vi "UpdateActualDepsList.vi"(8 "error in (no error)":errorcluster, 10 "UpdateForChangedLibrariesOnly":bool=TRUE, 11 "Workspace Path":path=path "C:/sw-deps-monitor") -> (0 "error out":errorcluster)   [LabVIEW 2019, in "Hawkeye.lvlib"]
uses:
  Hawkeye.lvlib
  <vilib>/Wiresmith Technology/G CLI/CLI Class/CLI.lvclass
  <vilib>/SLL Toolkit/SLL String/SLL String.lvlib
panel:
  in  "GUI Mode? {F)":bool
  in  "Tab Control":enum32{"GUI Mode", "CLI Mode"}(tab)
  out "Args":string[](array[string])=["C:\\sw-deps-monitor", "True"]
  out "Status Indicator":string
  # "When in GUI Mode, the controls will be used, \nIn CLI Mode, the Args will be used"
  # "Workspace Path"
  # "UpdateChangedLibsOnly? True/False"
  # "Command to run the VI from terminal\ng-cli -v --lv-ver 2023 --arch 32 \"C:\\sw-deps-monitor\\CICD\\AutomatedChecks\\UpdateActualDepsList.vi\" -- \"C:\\sw-deps-monitor\" \"False\""
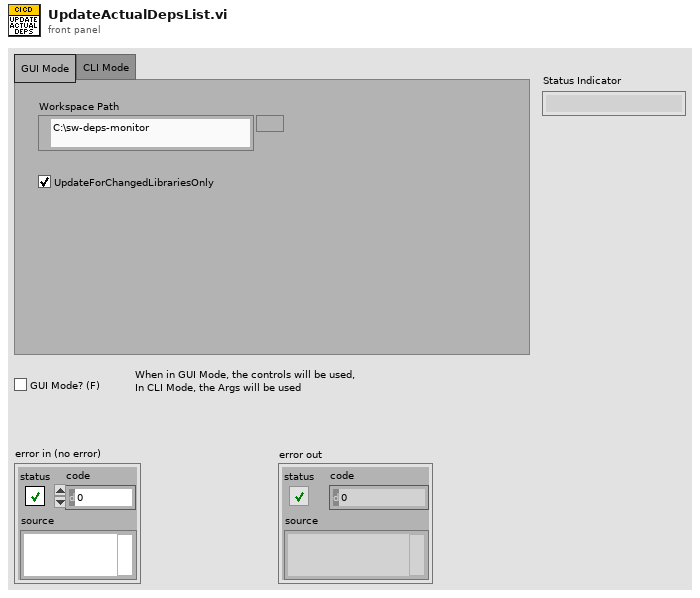
[diagram p1: front panel]
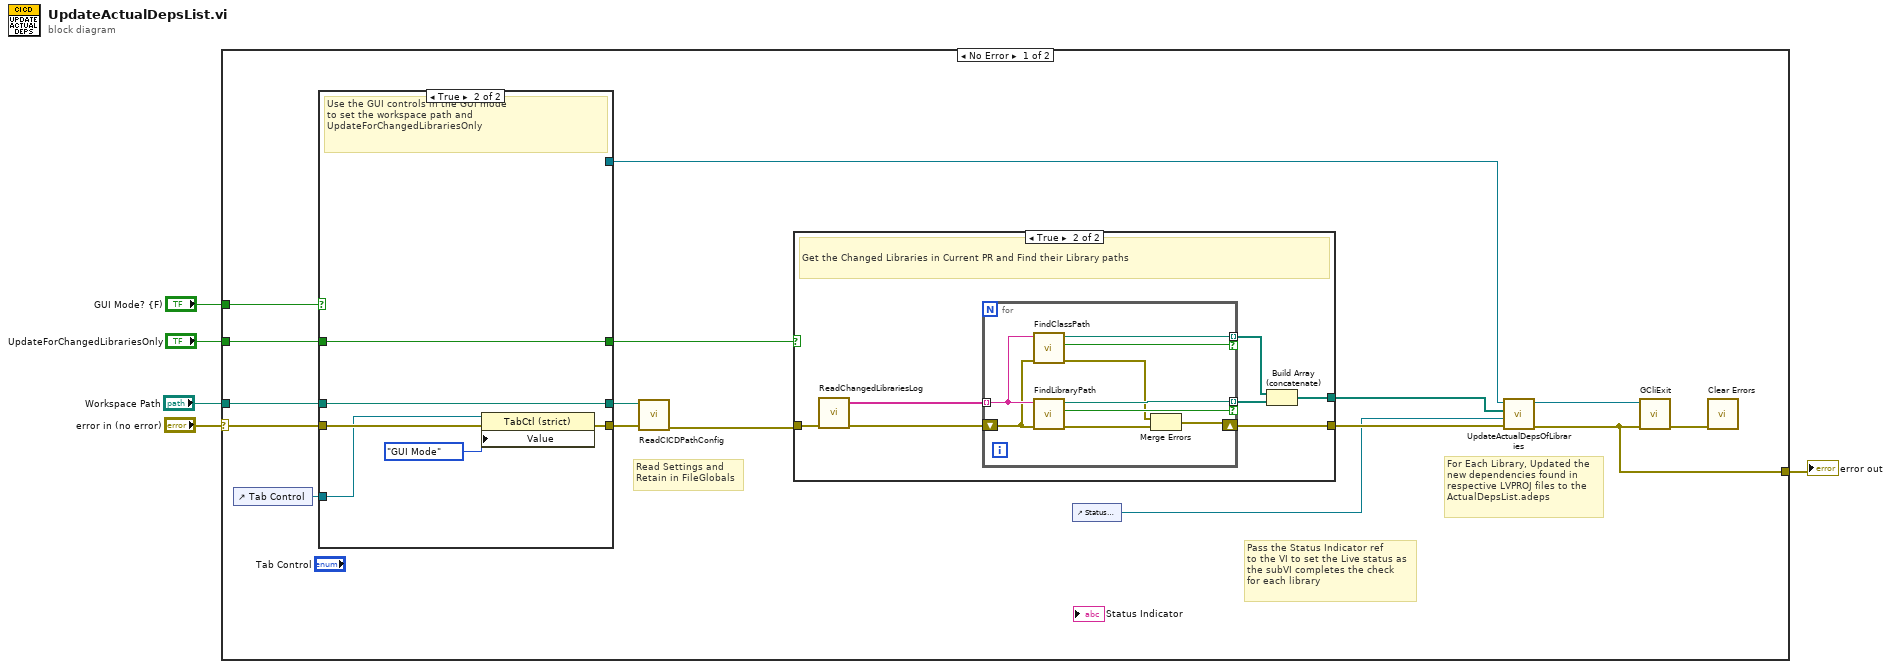
[diagram p0: block diagram]
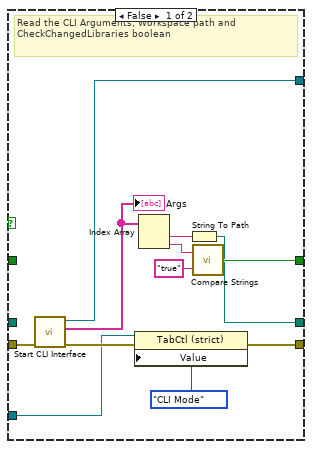
[diagram p2: hidden frame]
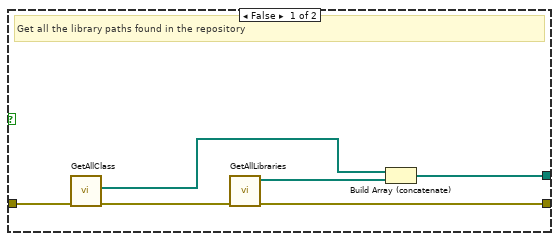
[diagram p3: hidden frame]
diagram:
  n1 = case shown="No Error" "error in (no error)" {
    selector: "error in (no error)" -> [w19 w62]
    tunnel: "GUI Mode? {F)" -> [w17 _]
    tunnel: [w11 w62] -> w3
    tunnel: "UpdateForChangedLibrariesOnly" -> [w7 _]
    tunnel: "Workspace Path" -> [w6 _]
    frame No Error {
      # "For Each Library, Updated the\nnew dependencies found in \nrespective LVPROJ files to the\nActualDepsList.adeps"
      # "Pass the Status Indicator ref\nto the VI to set the Live status as\nthe subVI completes the check\nfor each library"
      # "Read Settings and\nRetain in FileGlobals"
      n2 = control-ref of="Tab Control"() -> (w18:refnum<vi>)
      n3 = case shown="True" w17 {
        tunnel: w19 -> [w33 w39]
        tunnel: [w30 w38] -> w16
        tunnel: [w26 w35] -> w14
        tunnel: [w25 w34] -> w15
        tunnel: [w24 _] -> w13
        tunnel: w18 -> [w23 w36]
        tunnel: w7 -> [_ w35]
        tunnel: w6 -> [_ w34]
        frame False {
          # "Read the CLI Arguments, Workspace path and\nCheckChangedLibraries boolean"
          n4 = call <vilib>:"Start CLI Interface.vi"("error in (no error)"=w33) -> ("error out"=w32:errorcluster, "Custom Parameters"=w22:string[], "CLI out"=w24:refnum<class "CLI.lvclass">)  [unwired: 7 in, 1 out]
          "Args" <- w22
          n5 = property on="Property Node" class="TabCtl (strict)"(reference=w23, error in=w32, "Value"=enum32{"GUI Mode", "CLI Mode"}."CLI Mode" ("Tab Control")) -> (error out=w30:errorcluster)  [unwired: 1 out]
          n6 = Index Array(array=w22) -> (element #1=w29:string, element #2=w28:string)  [unwired: 2 in]
          n7 = String To Path(string=w29) -> (path=w25:path)
          n8 = call <vilib>:"Compare Strings.vi"("y"="true", "x"=w28) -> ("Equal?"=w26:bool)
        }
        frame True {
          # "Use the GUI controls in the GUI mode\nto set the workspace path and\nUpdateForChangedLibrariesOnly"
          n9 = property on="Property Node" class="TabCtl (strict)"(reference=w36, error in=w39, "Value"=enum32{"GUI Mode", "CLI Mode"}."GUI Mode" ("Tab Control")) -> (error out=w38:errorcluster)  [unwired: 1 out]
        }
      }
      n10 = call "ReadCICDPathConfig.vi"("error in (no error)"=w16, "Workspace Path"=w15) -> ("error out"=w20:errorcluster)  [unwired: 8 in, 1 out]
      n11 = case shown="True" w14 {
        tunnel: w20 -> [w41 w50]
        tunnel: [w43 w47] -> w9
        tunnel: [w44 w51] -> w21
        frame False {
          # "Get all the library paths found in the repository"
          n12 = call "GetAllClass.vi"("error in (no error)"=w41) -> ("error out"=w42:errorcluster, "Not owned (outside .lvlib)"=w40:path[])  [unwired: 7 in, 2 out]
          n13 = call "GetAllLibraries.vi"("error in (no error)"=w42) -> ("error out"=w44:errorcluster, "Lvlib paths"=w45:path[])  [unwired: 9 in]
          n14 = Build Array (concatenate)(w40, w45) -> (w43:path[])
        }
        frame True {
          # "Get the Changed Libraries in Current PR and Find their Library paths"
          n15 = call "ReadChangedLibrariesLog.vi"("error in (no error)"=w50) -> ("error out"=w49:errorcluster, "ChangedLibraries"=w48:string[])  [unwired: 9 in]
          n16 = for {
            tunnel: w48 -> [w58] mode=indexing
            shift-right: [w57] -> w51
            shift-left: w49 -> [w55]
            tunnel: [w60] -> w52 mode=indexing if=w59
            tunnel: [w54] -> w46 mode=indexing if=w53
            n17 = call "FindClassPath.vi"("error in (no error)"=w55, "Class Name"=w58) -> ("error out"=w56:errorcluster, "Found?"=w53:bool, "Library Path"=w54:path)  [unwired: 7 in]
            n18 = call "FindLibraryPath.vi"("error in (no error)"=w55, "Library Name"=w58) -> ("error out"=w61:errorcluster, "Found?"=w59:bool, "Library Path"=w60:path)  [unwired: 7 in]
            n19 = Merge Errors(w56, w61) -> (w57:errorcluster)
          }
          n20 = Build Array (concatenate)(w46, w52) -> (w47:path[])
        }
      }
      n21 = control-ref of="Status Indicator"() -> (w8:refnum<vi>)
      n22 = call "UpdateActualDepsOfLibraries.vi"("error in (no error)"=w21, "Status Indicator Ref"=w8, "Lvlib paths"=w9, "CLI in"=w13) -> ("error out"=w11:errorcluster, "CLI out"=w12:refnum<class "CLI.lvclass">)  [unwired: 6 in]
      n23 = call "GCliExit.vi"("error in (no error)"=w11, "CLI in"=w12) -> ("error out"=w10:errorcluster)  [unwired: 9 in]
      n24 = call <vilib>:"Clear Errors.vi"("error in (no error)"=w10) -> ()  [unwired: 5 in, 2 out]
    }
    frame Error {
    }
  }
  "error out" <- w3
